vi "VisitLVClusterType.vi"(8 "error in (no error)":errorcluster, 10 "LVClusterType":refnum<class "LVClusterType.lvclass">, 11 "NextGenXMLTypeGenerator in":refnum<class "NextGenXMLTypeGenerator.lvclass">) -> (0 "error out":errorcluster, 3 "NextGenXMLTypeGenerator out":refnum<class "NextGenXMLTypeGenerator.lvclass">)   [LabVIEW 2020, in "Web Service Description.lvlib" / "NextGenXMLTypeGenerator.lvclass"]
uses:
  <vilib>/AppBuilder/Engine/WebServiceDescription/NextGenXMLTypeGenerator/NextGenXMLTypeGenerator.lvclass
  e:/builds/penguin/labview/branches/2020/dev/dist/vi.lib/AppBuilder/Engine/WebServiceDescription/LVDataTypes/LVTypeVisitor/LVTypeVisitor.lvclass
  <vilib>/AppBuilder/Engine/WebServiceDescription/LVDataTypes/LVClusterType/LVClusterType.lvclass
  <vilib>/AppBuilder/Engine/WebServiceDescription/XMLGen/ValuePair.ctl
  <vilib>/AppBuilder/Engine/WebServiceDescription/NextGenXMLTypeGenerator/NextGenXMLTypeGenerator.lvclass/NextGenXMLTypeGenerator.ctl
  <vilib>/AppBuilder/Engine/WebServiceDescription/GetTypeAttributesVisitor/GetTypeAttributesVisitor.lvclass
  <vilib>/AppBuilder/Engine/WebServiceDescription/LVDataTypes/LVType/LVType.lvclass
  <vilib>/AppBuilder/Engine/WebServiceDescription/XMLGen/XMLGen.lvlib
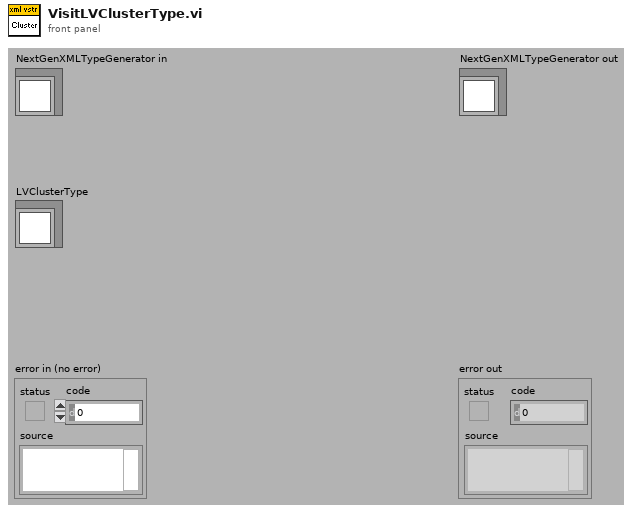
[diagram p1: front panel]
types:
  T1 = typedef "XMLGen.lvlib/ValuePair.ctl" = cluster{"Name":string, "Value":string}
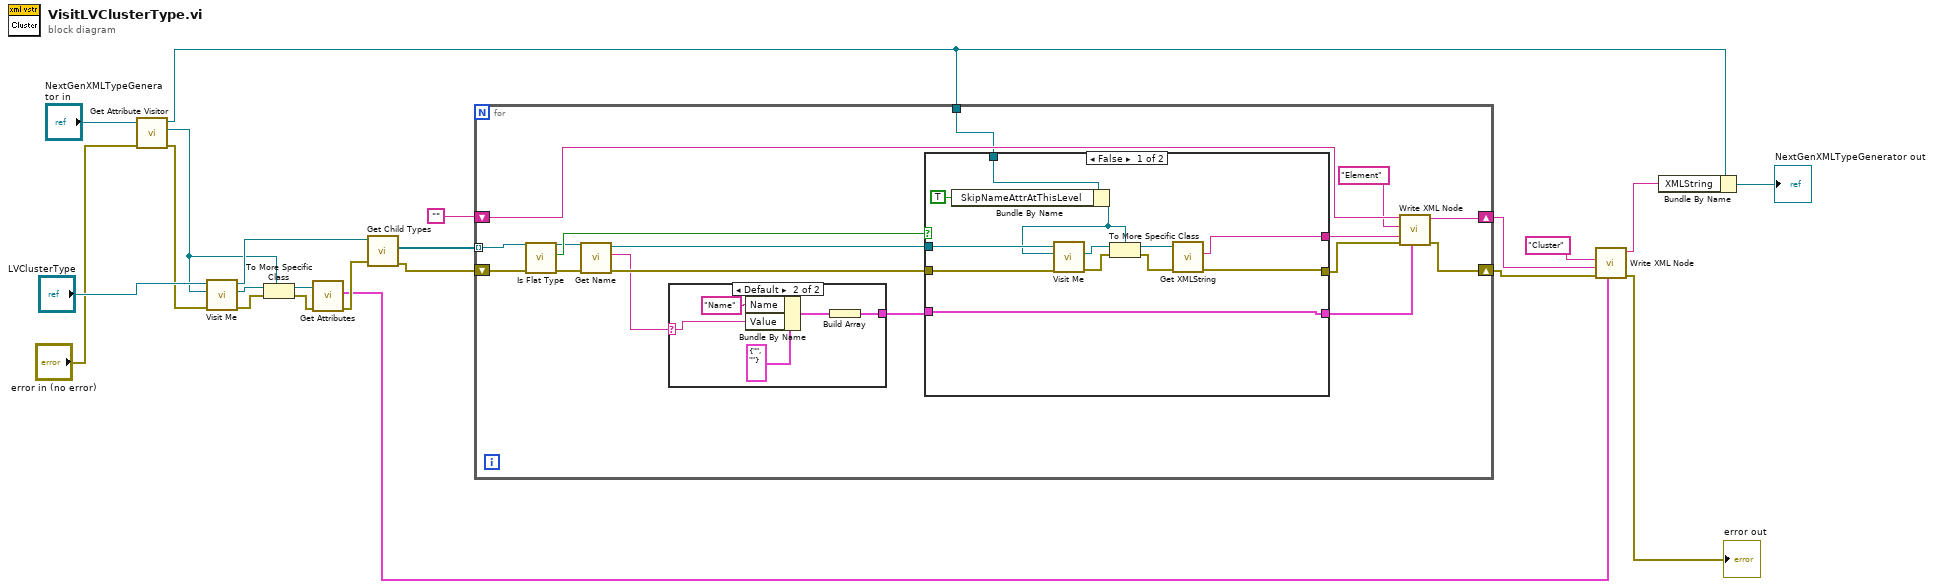
[diagram p0: block diagram]
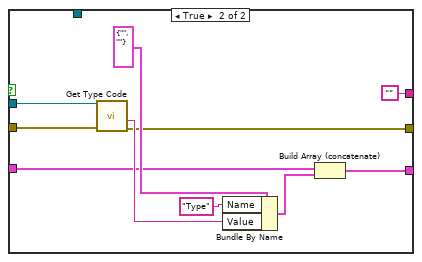
[diagram p3: hidden frame]
diagram:
  n1 = call <vilib>:"Get Attribute Visitor.vi"("error in (no error)"="error in (no error)", "NextGenXMLTypeGenerator in"="NextGenXMLTypeGenerator in") -> ("error out"=w3:errorcluster, "Attribute Visitor"=w2:refnum<class "GetTypeAttributesVisitor.lvclass">, "NextGenXMLTypeGenerator out"=w1:refnum<class "NextGenXMLTypeGenerator.lvclass">)  [unwired: 7 out]
  n2 = call-dynamic "Visit Me.vi"("error in (no error)"=w3, "Visitor In"=w2, "LVClusterType in"="LVClusterType") -> ("error out"=w12:errorcluster, "Visitor Out"=w13:refnum<class "LVTypeVisitor.lvclass">, "LVClusterType out"=w8:refnum<class "LVClusterType.lvclass">)  [unwired: 6 out]
  n3 = To More Specific Class(target class=w2, reference=w13, error in=w12) -> (specific class reference=w10:refnum<class "GetTypeAttributesVisitor.lvclass">, error out=w11:errorcluster)
  n4 = call <vilib>:"Get Attributes.vi"("error in (no error)"=w11, "GetTypeAttributesVisitor.lvclass in"=w10) -> ("error out"=w7:errorcluster, "Attributes"=w6:T1[])  [unwired: 8 out]
  n5 = call <vilib>:"Get Child Types.vi"("error in (no error)"=w7, "LVClusterType.lvclass in"=w8) -> ("error out"=w22:errorcluster, "Children"=w21:refnum<class "LVType.lvclass">[])  [unwired: 8 out]
  n6 = for {
    shift-right: [w26] -> w18
    shift-left: w22 -> [w38]
    tunnel: w21 -> [w39] mode=indexing
    shift-right: [w33] -> w17
    shift-left: "" -> [w34]
    tunnel: w1 -> [w25]
    n7 = call-dynamic "Is Flat Type.vi"("error in (no error)"=w38, "LVType in"=w39) -> ("error out"=w36:errorcluster, "Flat Type?"=w37:bool, "LVType out"=w35:refnum<class "LVType.lvclass">)  [unwired: 7 out]
    n8 = call <vilib>:"Get Name.vi"("error in (no error)"=w36, "LVType.lvclass in"=w35) -> ("error out"=w31:errorcluster, "Name"=w24:string, "LVType.lvclass out"=w30:refnum<class "LVType.lvclass">)  [unwired: 7 out]
    n9 = case shown="Default" w24 {
      selector: w24 -> [_ w40]
      tunnel: [_ w41] -> w23
      frame "" {
      }
      frame Default {
        n10 = Bundle By Name(cluster=T1 {"Name"="", "Value"=""} ("Attribute"), "Name"="Name", "Value"=w40) -> (w43:T1)
        n11 = Build Array(w43) -> (w41:T1[])
      }
    }
    n12 = case shown="False" w37 {
      tunnel: w23 -> [w48 w57]
      tunnel: w31 -> [w55 w64]
      tunnel: w30 -> [w56 w63]
      tunnel: [w48 w60] -> w29
      tunnel: [w49 w59] -> w28
      tunnel: [w50 ""] -> w27
      tunnel: w25 -> [w47 _]
      frame False {
        n13 = Bundle By Name(cluster=w47, "SkipNameAttrAtThisLevel"=TRUE) -> (w45:refnum<class "NextGenXMLTypeGenerator.lvclass">)
        n14 = call-dynamic "Visit Me.vi"("error in (no error)"=w55, "Visitor In"=w45, "LVType in"=w56) -> ("error out"=w53:errorcluster, "Visitor Out"=w54:refnum<class "LVTypeVisitor.lvclass">)  [unwired: 7 out]
        n15 = To More Specific Class(target class=w45, reference=w54, error in=w53) -> (specific class reference=w51:refnum<class "NextGenXMLTypeGenerator.lvclass">, error out=w52:errorcluster)
        n16 = call <vilib>:"Get XMLString.vi"("error in (no error)"=w52, "NextGenXMLTypeGenerator.lvclass in"=w51) -> ("error out"=w49:errorcluster, "XMLString"=w50:string)  [unwired: 8 out]
      }
      frame True {
        n17 = call <vilib>:"Get Type Code.vi"("error in (no error)"=w64, "LVType.lvclass in"=w63) -> ("error out"=w59:errorcluster, "TypeCodeString"=w62:string)  [unwired: 8 out]
        n18 = Bundle By Name(cluster=T1 {"Name"="", "Value"=""} ("Attribute"), "Name"="Type", "Value"=w62) -> (w61:T1)
        n19 = Build Array (concatenate)(w57, w61) -> (w60:T1[])
      }
    }
    n20 = call <vilib>:"Write XML Node.vi"("attributes"=w29, "error in (no error)"=w28, "body"=w27, "node"="Element", "initial string"=w34) -> ("error out"=w26:errorcluster, "resulting string"=w33:string)  [unwired: 5 out]
  }
  n21 = call <vilib>:"Write XML Node.vi"("attributes"=w6, "error in (no error)"=w18, "body"=w17, "node"="Cluster") -> ("error out"=→"error out":errorcluster, "resulting string"=w15:string)  [unwired: 1 in, 5 out]
  n22 = Bundle By Name(cluster=w1, "XMLString"=w15) -> (→"NextGenXMLTypeGenerator out":refnum<class "NextGenXMLTypeGenerator.lvclass">)
